vi "ReadbyWeakRefBool.vi"(8 "error in":errorcluster caption="entrée d'erreur", 11 "Control Ref":refnum<vi>) -> (0 "error out":errorcluster caption="sortie d'erreur", 3 "Valeur":bool)   [LabVIEW 2012]
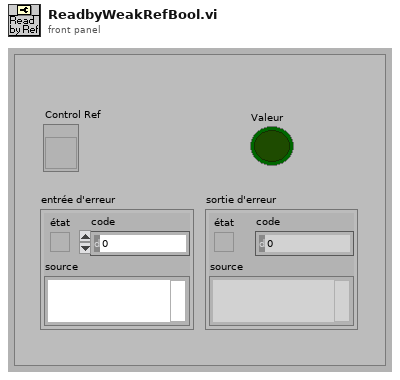
[diagram p1: front panel]
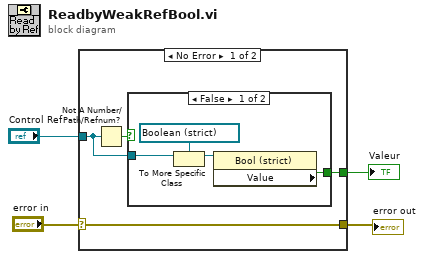
[diagram p0: block diagram]
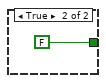
[diagram p2: hidden frame]
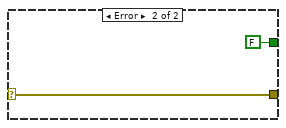
[diagram p3: hidden frame]
diagram:
  n1 = case shown="No Error" "error in" {
    selector: "error in" -> [w5 w15]
    tunnel: "Control Ref" -> [w7 _]
    tunnel: [w6 FALSE ("Value")] -> w3
    tunnel: [w5 w15] -> w1
    frame No Error {
      n2 = Not A Number/Path/Refnum?(number/path/refnum=w7) -> (NaN/Path/Refnum?=w8:bool)
      n3 = case shown="False" w8 {
        tunnel: w7 -> [w10 _]
        tunnel: [w12 FALSE ("Value")] -> w6
        frame False {
          n4 = To More Specific Class(target class=refnum<vi> refnum ("MovingRef"), reference=w10) -> (specific class reference=w9:refnum<vi>)  [unwired: 1 in, 1 out]
          n5 = property class="Bool (strict)"(reference=w9) -> ("Value"=w12:bool)  [unwired: 1 in, 2 out]
        }
        frame True {
        }
      }
    }
    frame Error {
    }
  }
  "Valeur" <- w3
  "error out" <- w1
